vi "PPL_NET_Test.vi"() -> ()   [LabVIEW 2018]
uses:
  builds/HTTP REST NET/LabVIEWHTTPClient_NET PPL/LabVIEWHTTPClient_NET.lvlibp/Types/method_enum.ctl
  builds/HTTP REST NET/LabVIEWHTTPClient_NET PPL/LabVIEWHTTPClient_NET.lvlibp/LabVIEWHTTPClient_NET/LabVIEWHTTPClient_NET.lvclass
  builds/HTTP REST NET/LabVIEWHTTPClient_NET PPL/LabVIEWHTTPClient_NET.lvlibp
  builds/HTTP REST NET/LabVIEWHTTPClient_NET PPL/LabVIEWHTTPClient_NET.lvlibp/WebProxy_NET/WebProxy_NET.lvclass
panel:
  in  "Array - String":string[](array[string])=["https://reqres.in/api/users?page=2", "http://redmine.viviota.com:8005/ActivationServer/ping", "https://maps.googleapis.com/maps/api/streetview/metadata?size=600x300&location=eiffel%20tower,%20paris,%20france&heading=-45&pitch=42&fov=110&key=AIzaSyDuYQg9m45HZeNlFCN-9AhsuZy1Uii3f18"]
  out "StatusCode":i32(ring)=100 items=["Continue"=100, "SwitchingProtocols"=101, "OK"=200, "Created"=201, "Accepted"=202, "NonAuthoritativeInformation"=203, "NoContent"=204, "ResetContent"=205, "PartialContent"=206, "MultipleChoices, Ambiguous"=300, "MovedPermanently, Moved"=301, "Found, Redirect"=302, "SeeOther, RedirectMethod"=303, "NotModified"=304, "UseProxy"=305, "Unused"=306, "TemporaryRedirect, RedirectKeepVerb"=307, "BadRequest"=400, "Unauthorized"=401, "PaymentRequired"=402, "Forbidden"=403, "NotFound"=404, "MethodNotAllowed"=405, "NotAcceptable"=406, "ProxyAuthenticationRequired"=407, "RequestTimeout"=408, "Conflict"=409, "Gone"=410, "LengthRequired"=411, "PreconditionFailed"=412, "RequestEntityTooLarge"=413, "RequestUriTooLong"=414, "UnsupportedMediaType"=415, "RequestedRangeNotSatisfiable"=416, "ExpectationFailed"=417, "UpgradeRequired"=426, "InternalServerError"=500, "NotImplemented"=501, "BadGateway"=502, "ServiceUnavailable"=503, "GatewayTimeout"=504, "HttpVersionNotSupported"=505]
  in  "Proxy":string
  out "Response":string
  in  "URL":string
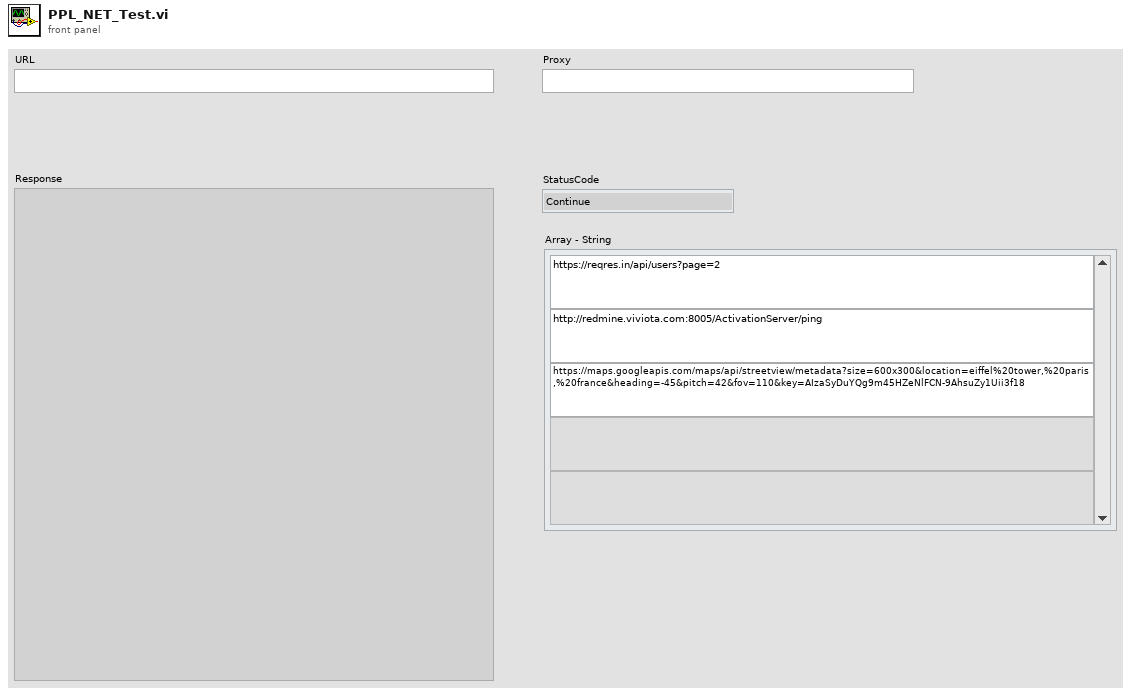
[diagram p1: front panel]
types:
  T1 = typedef "LabVIEWHTTPClient_NET.lvlibp/method_enum.ctl" = enum16{"GET", "PUT", "POST", "DELETE", "HEAD", "TRACE", "SEND"}
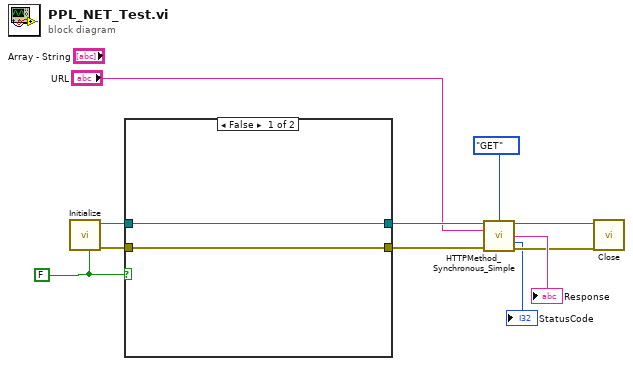
[diagram p0: block diagram]
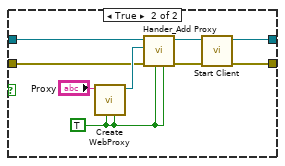
[diagram p2: hidden frame]
diagram:
  w8 = FALSE ("Allow Handler Configuration")
  n1 = call "Initialize.vi"("Allow Handler Configuration [F]"=w8) -> ("error out"=w5:errorcluster, "HTTP Client Out"=w7:refnum<class "LabVIEWHTTPClient_NET.lvclass">)  [unwired: 9 in]
  n2 = case shown="False" w8 {
    tunnel: w7 -> [w13 w22]
    tunnel: [w13 w20] -> w6
    tunnel: w5 -> [w12 w16]
    tunnel: [w12 w14] -> w4
    frame False {
    }
    frame True {
      w18 = TRUE ("UseDefaultCredentials [T]")
      n3 = call "Create WebProxy.vi"("BypassProxyOnLocal"=w18, "UseDefaultCredentials [T]"=w18, "Host"="Proxy") -> ("WebProxy Out"=w19:refnum<class "WebProxy_NET.lvclass">)  [unwired: 8 in]
      n4 = call "Hander_Add Proxy.vi"("PreAuthenticate"=w18, "UseProxy"=w18, "error in (no error)"=w16, "WebProxy"=w19, "LabVIEWHTTPClient_NET in"=w22) -> ("error out"=w15:errorcluster, "LabVIEWHTTPClient_NET out"=w21:refnum<class "LabVIEWHTTPClient_NET.lvclass">)  [unwired: 5 in]
      n5 = call "Start Client.vi"("error in (no error)"=w15, "LabVIEWHTTPClient_NET in"=w21) -> ("error out"=w14:errorcluster, "LabVIEWHTTPClient_NET out"=w20:refnum<class "LabVIEWHTTPClient_NET.lvclass">)  [unwired: 8 in]
    }
  }
  n6 = call "HTTPMethod_Synchronous_Simple.vi"("LabVIEWHTTPClient_NET in"=w6, "Method"=method_enum."GET", "URL"="URL", "error in (no error)"=w4) -> ("LabVIEWHTTPClient_NET out"=w11:refnum<class "LabVIEWHTTPClient_NET.lvclass">, "Response"=→"Response":string, "StatusCode"=→"StatusCode":i32, "error out"=w2:errorcluster)  [unwired: 6 in, 2 out]
  n7 = call "Close.vi"("error in (no error)"=w2, "LabVIEWHTTPClient_NET in"=w11) -> ()  [unwired: 9 in, 1 out]
